vi "Write Log File.vi"(8 "error in (no error)":errorcluster, 9 "Message In":string, 10 "Filename In":string, 11 "File Path In":path) -> (3 "FilePath out":path)   [LabVIEW 2024, in "LVarex.lvlib"]
uses:
  LVarex.lvlib
panel:
  out "error out":errorcluster
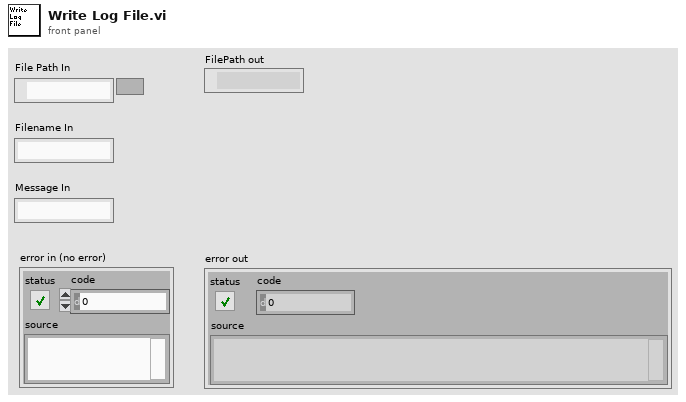
[diagram p1: front panel]
types:
  T1 = enum16{"open", "replace", "create", "open or create", "replace or create", "replace or create with confirmation"}
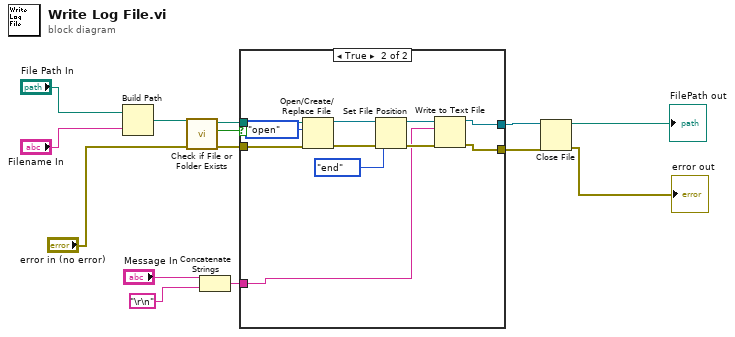
[diagram p0: block diagram]
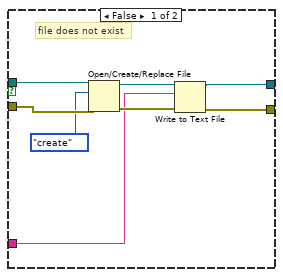
[diagram p2: hidden frame]
diagram:
  n1 = Build Path(base path="File Path In", name or relative path="Filename In") -> (appended path=w12:path)
  n2 = call <vilib>:"Check if File or Folder Exists.vi"("error in (no error)"="error in (no error)", "path"=w12) -> ("error out"=w8:errorcluster, "file or folder exists?"=w10:bool, "dup path"=w9:path)  [unwired: 7 in]
  n3 = Concatenate Strings("Message In", "\r\n") -> (w5:string)
  n4 = case shown="True" w10 {
    tunnel: w9 -> [w22 w33]
    tunnel: w8 -> [w21 w32]
    tunnel: w5 -> [w17 w25]
    tunnel: [w16 w24] -> w4
    tunnel: [w15 w23] -> w3
    frame False {
      # "file does not exist"
      n5 = Open/Create/Replace File(file path (use dialog)=w22, error in=w21, operation (0:open)=T1."create") -> (refnum out=w19:refnum<file>, error out=w18:errorcluster)  [unwired: 3 in, 1 out]
      n6 = Write to Text File(file (use dialog)=w19, text=w17, error in=w18) -> (refnum out=w16:refnum<file>, error out=w15:errorcluster)  [unwired: 1 in, 1 out]
    }
    frame True {
      n7 = Open/Create/Replace File(file path (use dialog)=w33, error in=w32, operation (0:open)=T1."open") -> (refnum out=w30:refnum<file>, error out=w29:errorcluster)  [unwired: 3 in, 1 out]
      n8 = Set File Position(refnum=w30, from (0:start)=enum16{"start", "end", "current"}."end", error in=w29) -> (refnum out=w26:refnum<file>, error out=w27:errorcluster)  [unwired: 1 in]
      n9 = Write to Text File(file (use dialog)=w26, text=w25, error in=w27) -> (refnum out=w24:refnum<file>, error out=w23:errorcluster)  [unwired: 1 in, 1 out]
    }
  }
  n10 = Close File(refnum=w4, error in=w3) -> (path=→"FilePath out":path, error out=→"error out":errorcluster)
